vi "Final_UI.vi"() -> ()   [LabVIEW 2020]
panel:
  in  "VISA resource name":refnum<visa-resource-name>
  out "Humiditty 2":dbl(graph)
  out "Temp 3":dbl(graph)
  out "Humidity 2":dbl(knob) scale=0.0..10.0
  out "Temp 2":dbl(slide) scale=0.0..50.0
  in  "Table Control":string[][](table)
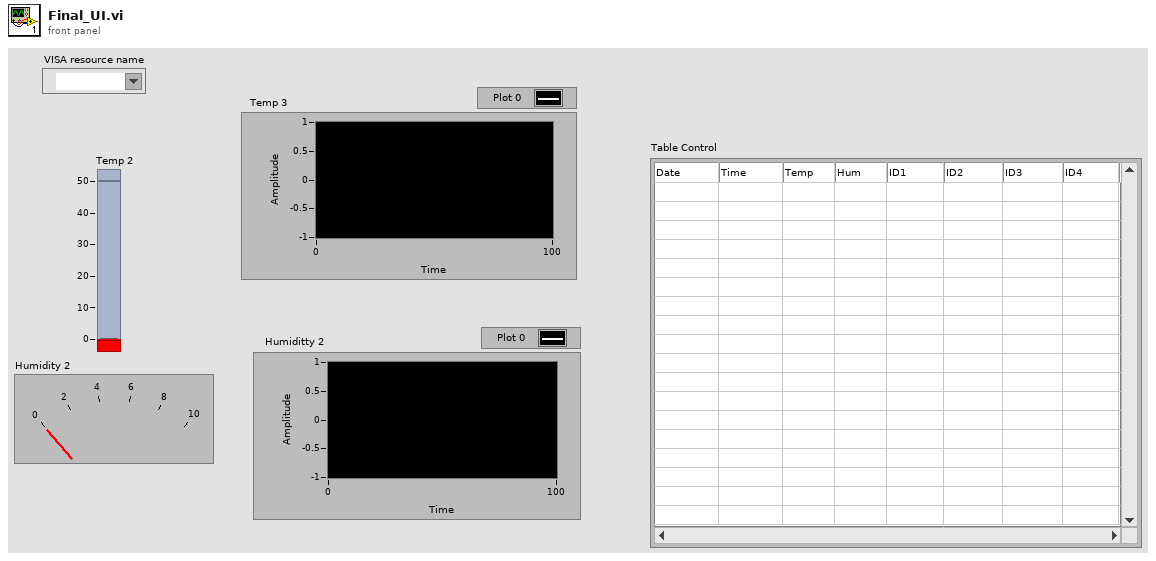
[diagram p1: front panel]
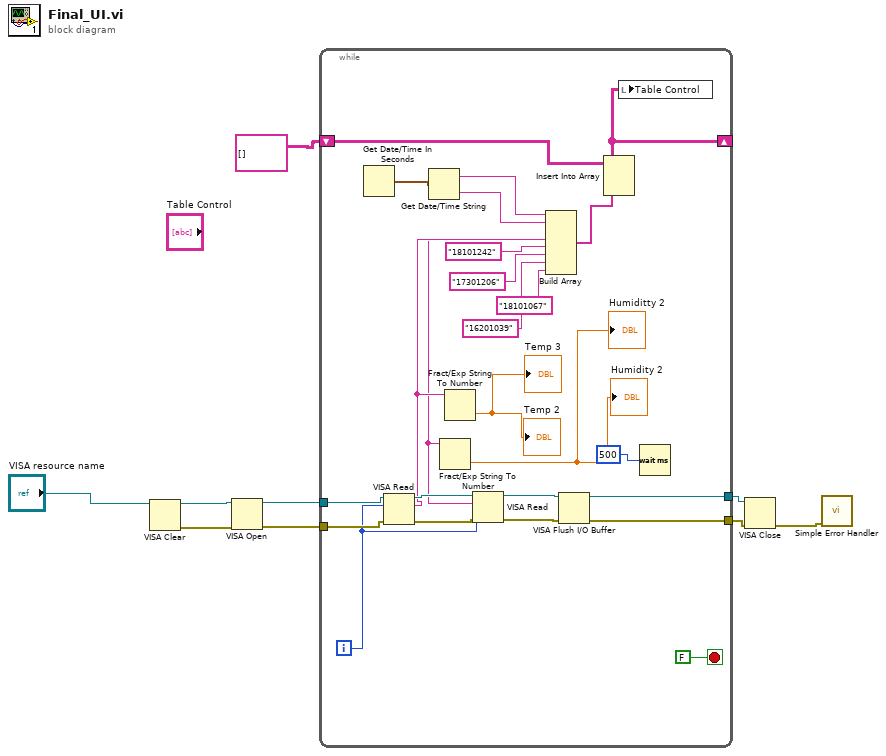
[diagram p0: block diagram]
diagram:
  n1 = VISA Clear(VISA resource name="VISA resource name") -> (VISA resource name out=w9:refnum<visa-resource-name>, error out=w8:errorcluster)  [unwired: 1 in]
  n2 = VISA Open(error in (no error)=w8, VISA resource name=w9) -> (VISA resource name=w7:refnum<visa-resource-name>, error out=w6:errorcluster)  [unwired: 3 in]
  n3 = while {
    tunnel: w7 -> [w34]
    tunnel: w6 -> [w33]
    tunnel: [w29] -> w5
    tunnel: [w28] -> w4
    shift-right: [w24] -> _
    shift-left: string[][] [] -> [w25]
    i -> [w27]
    stop <- FALSE stop-if-true
    n4 = Get Date/Time In Seconds() -> (seconds since 1Jan1904=w20:timestamp)
    n5 = VISA Read(VISA resource name=w34, byte count=w27, error in (no error)=w33) -> (VISA resource name out=w23:refnum<visa-resource-name>, read buffer=w17:string, error out=w32:errorcluster)  [unwired: 1 out]
    n6 = Get Date/Time String(seconds (now)=w20) -> (date string=w19:string, time string=w18:string)  [unwired: 2 in]
    n7 = Fract/Exp String To Number(string=w17) -> (number=→"Temp 2" →"Temp 3":dbl)  [unwired: 3 in, 1 out]
    n8 = VISA Read(VISA resource name=w23, byte count=w27, error in (no error)=w32) -> (VISA resource name out=w31:refnum<visa-resource-name>, read buffer=w16:string, error out=w30:errorcluster)  [unwired: 1 out]
    n9 = Fract/Exp String To Number(string=w16) -> (number=→"Humidity 2" →"Humiditty 2":dbl)  [unwired: 3 in, 1 out]
    n10 = Build Array(w19, w18, w17, w16, "18101242" ("element"), "17301206" ("element"), "16201039" ("element"), "18101067" ("element")) -> (w14:string[])
    n11 = VISA Flush I/O Buffer(VISA resource name=w31, error in (no error)=w30) -> (VISA resource name out=w29:refnum<visa-resource-name>, error out=w28:errorcluster)  [unwired: 1 in]
    n12 = Insert Into Array(array=w25, new element=w14) -> (w24:string[][])  [unwired: 2 in]
    n13 = local write "Table Control"(w24) -> ()
    n14 = Wait (ms)(milliseconds to wait=u32 500) -> ()  [unwired: 1 out]
  }
  n15 = VISA Close(VISA resource name=w5, error in (no error)=w4) -> (error out=w3:errorcluster)
  n16 = call <vilib>:"Simple Error Handler.vi"("error in (no error)"=w3) -> ()  [unwired: 4 in, 5 out]
